vi "1_3.vi"() -> ()   [LabVIEW 2020]
panel:
  out "Days":dbl
  out "Weeks":dbl
  out "Hours":dbl
  out "Minutes":dbl
  out "Seconds":dbl
  in  "Seconds":dbl
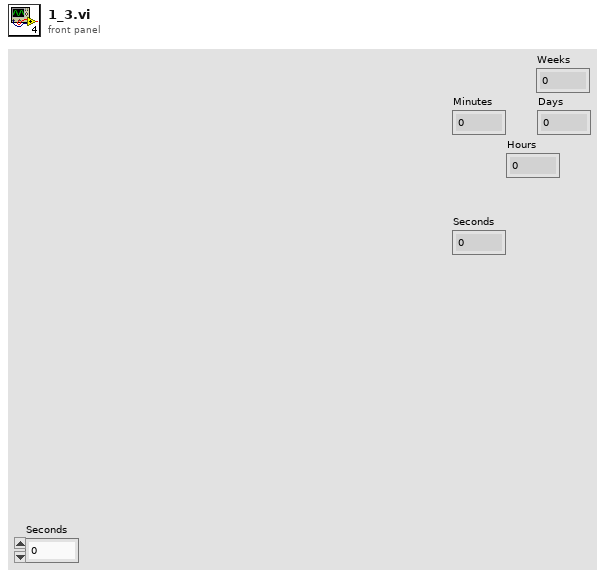
[diagram p1: front panel]
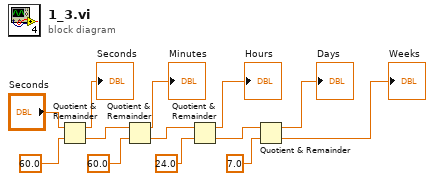
[diagram p0: block diagram]
diagram:
  n1 = Quotient & Remainder(x="Seconds", y=60.0) -> (x-y*floor(x/y)=→"Seconds":dbl, floor(x/y)=w8:dbl)
  n2 = Quotient & Remainder(x=w8, y=60.0) -> (x-y*floor(x/y)=→"Minutes":dbl, floor(x/y)=w6:dbl)
  n3 = Quotient & Remainder(x=w6, y=24.0) -> (x-y*floor(x/y)=→"Hours":dbl, floor(x/y)=w2:dbl)
  n4 = Quotient & Remainder(x=w2, y=7.0) -> (x-y*floor(x/y)=→"Days":dbl, floor(x/y)=→"Weeks":dbl)
